vi "labview side.vi"() -> ()   [LabVIEW 2023]
uses:
  <vilib>/Instr/_visa.llb/VISA Configure Serial Port (Instr).vi
panel:
  out "¤ô±Kªù":bool
  in  "2":bool
  in  "1":bool
  out "¤ô¦ì°ª«×":dbl(slide) scale=0.0..400.0
  in  "ֹͣ":bool
  out "Âà³tR.P.M":dbl(knob) scale=0.0..250.0
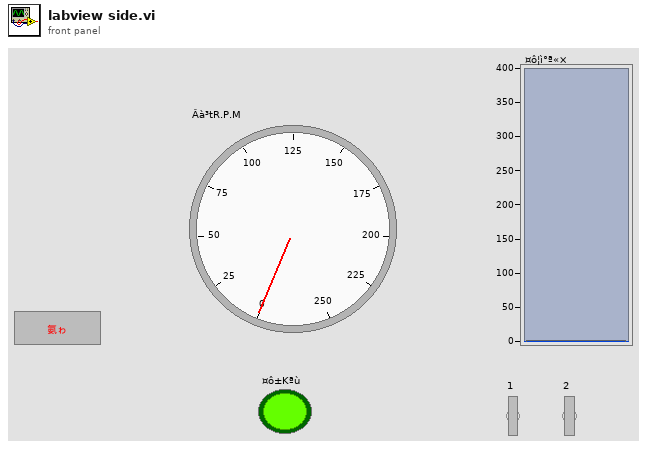
[diagram p1: front panel]
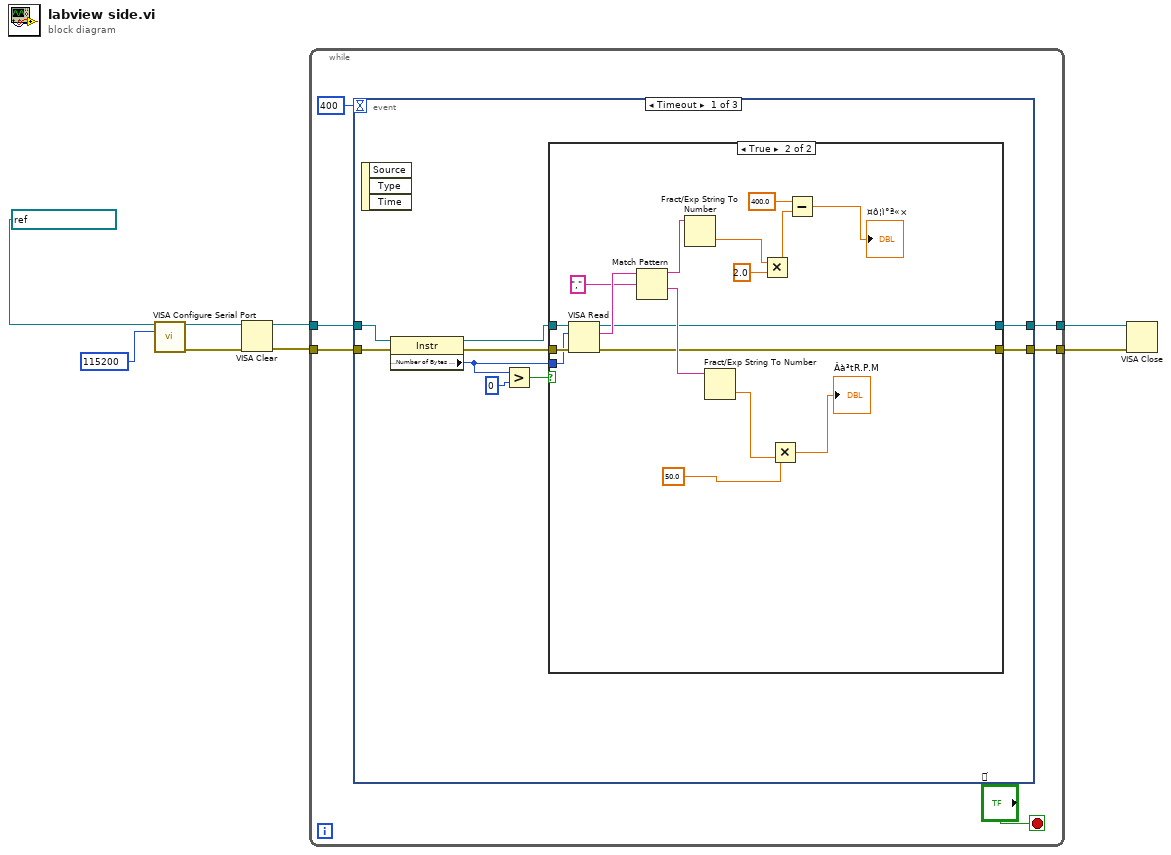
[diagram p0: block diagram]
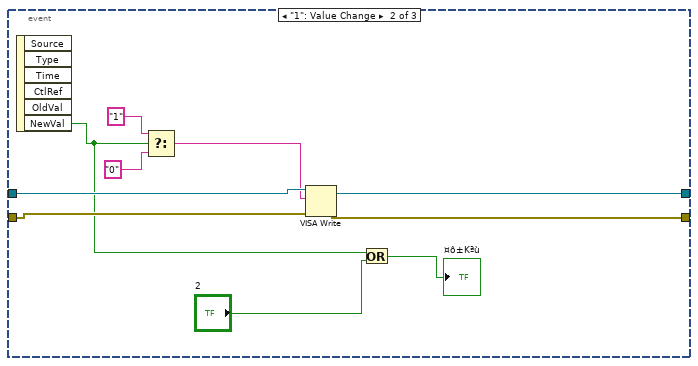
[diagram p3: hidden frame]
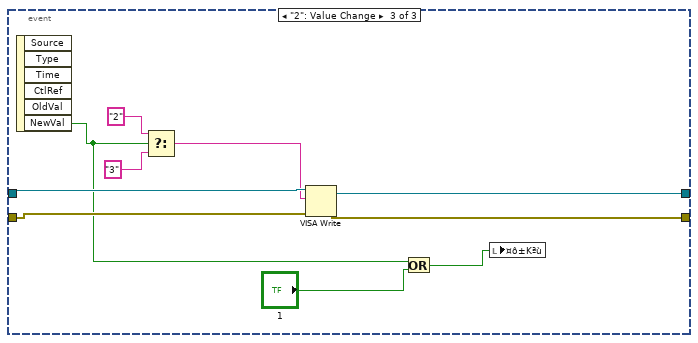
[diagram p4: hidden frame]
diagram:
  n1 = call-poly "VISA Configure Serial Port"("VISA resource name"=refnum<visa-resource-name> "ASRL5::INSTR" ("COM"), "baud rate (9600)"=115200) -> ("VISA resource name out"=w7:refnum<visa-resource-name>, "error out"=w3:errorcluster)  [unwired: 12 in]
  n2 = VISA Clear(VISA resource name=w7, error in (no error)=w3) -> (VISA resource name out=w4:refnum<visa-resource-name>, error out=w2:errorcluster)
  n3 = while {
    tunnel: w2 -> [w11]
    tunnel: [w13] -> w5
    tunnel: w4 -> [w12]
    tunnel: [w14] -> w6
    stop <- "ֹͣ" stop-if-true
    n4 = event shown="[0] Timeout" {
      selector: _ -> [_ _ _]
      dyn-events: _ -> [_ _ _]
      timeout: 400 -> [_ _ _]
      tunnel: [w23 w49 w59] -> w14
      tunnel: [w22 w50 w60] -> w13
      tunnel: w12 -> [w16 w52 w62]
      tunnel: w11 -> [w15 w51 w61]
      event Timeout {
        n5 = event-data() -> ()  [unwired: 1 in, 3 out]
        n6 = property class="Instr"(reference=w16, error in=w15) -> (reference out=w21:refnum<visa-resource-name>, error out=w20:errorcluster, "Serial Settings:Number of Bytes at Serial Port"=w17:u32)
        n7 = Greater?(x=w17, y=u32 0) -> (0:w18:bool)
        n8 = case shown="True" w18 {
          tunnel: [w24 w34] -> w22
          tunnel: [w25 w35] -> w23
          tunnel: w21 -> [w25 w42]
          tunnel: w20 -> [w24 w41]
          tunnel: w17 -> [_ w40]
          frame False {
          }
          frame True {
            n9 = VISA Read(VISA resource name=w42, byte count=w40, error in (no error)=w41) -> (VISA resource name out=w35:refnum<visa-resource-name>, read buffer=w39:string, error out=w34:errorcluster)  [unwired: 1 out]
            n10 = Match Pattern(string=w39, regular expression="," ("正则表达式")) -> (before substring=w36:string, after substring=w37:string)  [unwired: 1 in, 2 out]
            n11 = Fract/Exp String To Number(string=w36) -> (number=w28:dbl)  [unwired: 3 in, 1 out]
            n12 = Fract/Exp String To Number(string=w37) -> (number=w33:dbl)  [unwired: 3 in, 1 out]
            n13 = Multiply(x=w28, y=2.0) -> (x*y=w26:dbl)
            n14 = Multiply(x=50.0, y=w33) -> (x*y=→"Âà³tR.P.M":dbl)
            n15 = Subtract(x=400.0, y=w26) -> (x-y=→"¤ô¦ì°ª«×":dbl)
          }
        }
      }
      event "1": Value Change {
        n16 = event-data() -> ("NewVal"=w45:bool)  [unwired: 1 in, 5 out]
        n17 = Select(t="1", s=w45, f="0") -> (s? t:f=w46:string)
        n18 = VISA Write(VISA resource name=w52, write buffer=w46, error in (no error)=w51) -> (VISA resource name out=w49:refnum<visa-resource-name>, error out=w50:errorcluster)  [unwired: 1 out]
        n19 = Or(x=w45, y="2") -> (x .or. y?=→"¤ô±Kªù":bool)
      }
      event "2": Value Change {
        n20 = event-data() -> ("NewVal"=w55:bool)  [unwired: 1 in, 5 out]
        n21 = Select(t="2", s=w55, f="3") -> (s? t:f=w56:string)
        n22 = VISA Write(VISA resource name=w62, write buffer=w56, error in (no error)=w61) -> (VISA resource name out=w59:refnum<visa-resource-name>, error out=w60:errorcluster)  [unwired: 1 out]
        n23 = Or(x=w55, y="1") -> (x .or. y?=w53:bool)
        n24 = local write "¤ô±Kªù"(w53) -> ()
      }
    }
  }
  n25 = VISA Close(VISA resource name=w6, error in (no error)=w5) -> ()  [unwired: 1 out]
